vi "loadBoard.vi"(8 "error in (no error)":errorcluster, 10 "continuous":bool, 11 "SpinCore in":refnum<class "SpinCore.lvclass">) -> (0 "error out":errorcluster, 3 "SpinCore out":refnum<class "SpinCore.lvclass">)   [LabVIEW 2011, in "Hardware.lvlib" / "Channels.lvlib" / "SpinCore.lvclass"]
uses:
  SpinCore.lvclass
  SpinCore.lvclass/SpinCore.ctl
panel:
  out "Instructions":T1(array[cluster]) {"Op Code" items=["Continue", "Stop", "Loop", "End Loop", "JSR", "RTS", "Branch", "Long Delay", "Wait"]; "Amp Register2" items=["0", "1", "2", "3"]; "Phase Register2" items=["0", "1", "2", "3", "4", "5", "6", "7", "8", "9", "10", "11", "12", "13", "14", "15"]; "Freq Register2" items=["0", "1", "2", "3", "4", "5", "6", "7", "8", "9", "10", "11", "12", "13", "14", "15"]; "Amp Register1" items=["0", "1", "2", "3"]; "Phase Register1" items=["0", "1", "2", "3", "4", "5", "6", "7", "8", "9", "10", "11", "12", "13", "14", "15"]; "Freq Register1" items=["0", "1", "2", "3", "4", "5", "6", "7", "8", "9", "10", "11", "12", "13", "14", "15"]; "Length" format="%.6p"}
  out "dataChannel1":dbl[][](array[numeric])
  out "dataChannel0":dbl[][](array[numeric])
  # "0"
  # "1"
  # "2"
  # "3"
  # "4"
  # "5"
  # "6"
  # "7"
  # "8"
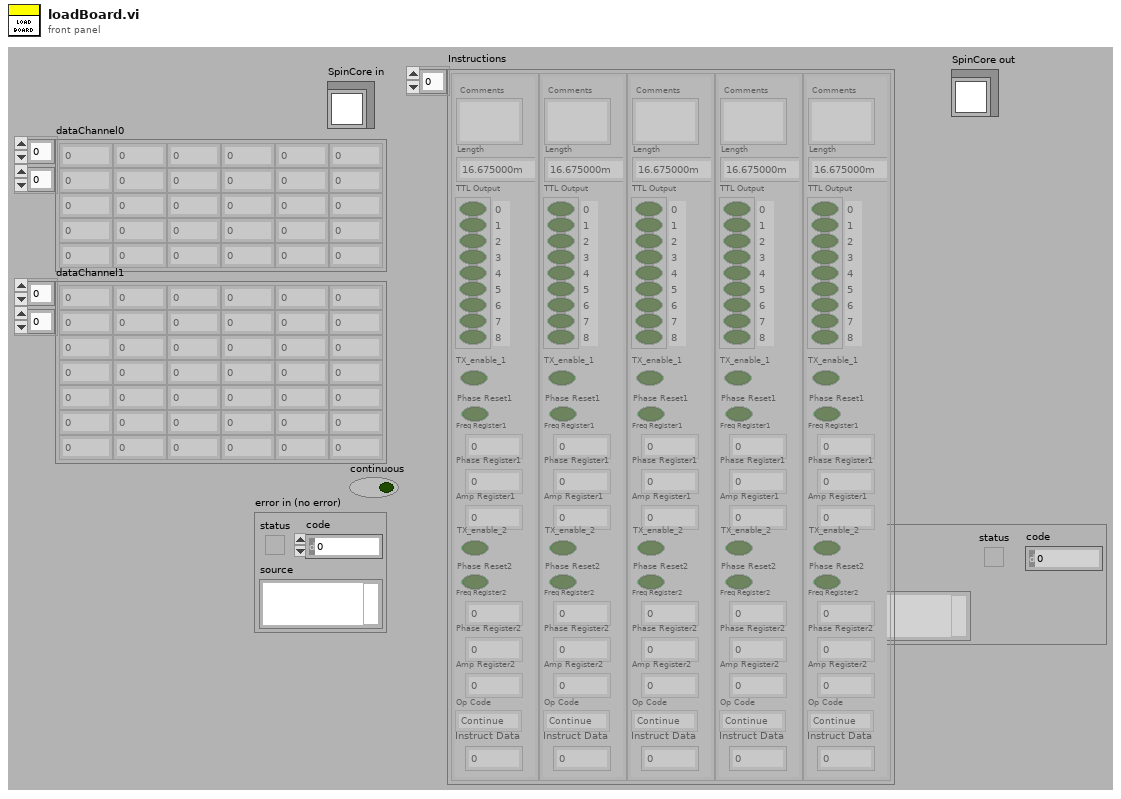
[diagram p1: front panel]
types:
  T1 = cluster{"Comments":string, "Length":dbl, "TTL Output":bool[], "TX_enable_1":bool, "Phase Reset1":bool, "Freq Register1":i32, "Phase Register1":i32, "Amp Register1":i32, "TX_enable_2":bool, "Phase Reset2":bool, "Freq Register2":i32, "Phase Register2":i32, "Amp Register2":i32, "Instruct Data":i32, "Op Code":i32}[]
  T2 = enum16{"Pulse Program", "Frequency Registers", "TX Phase Registers", "RX Phase Registers"}
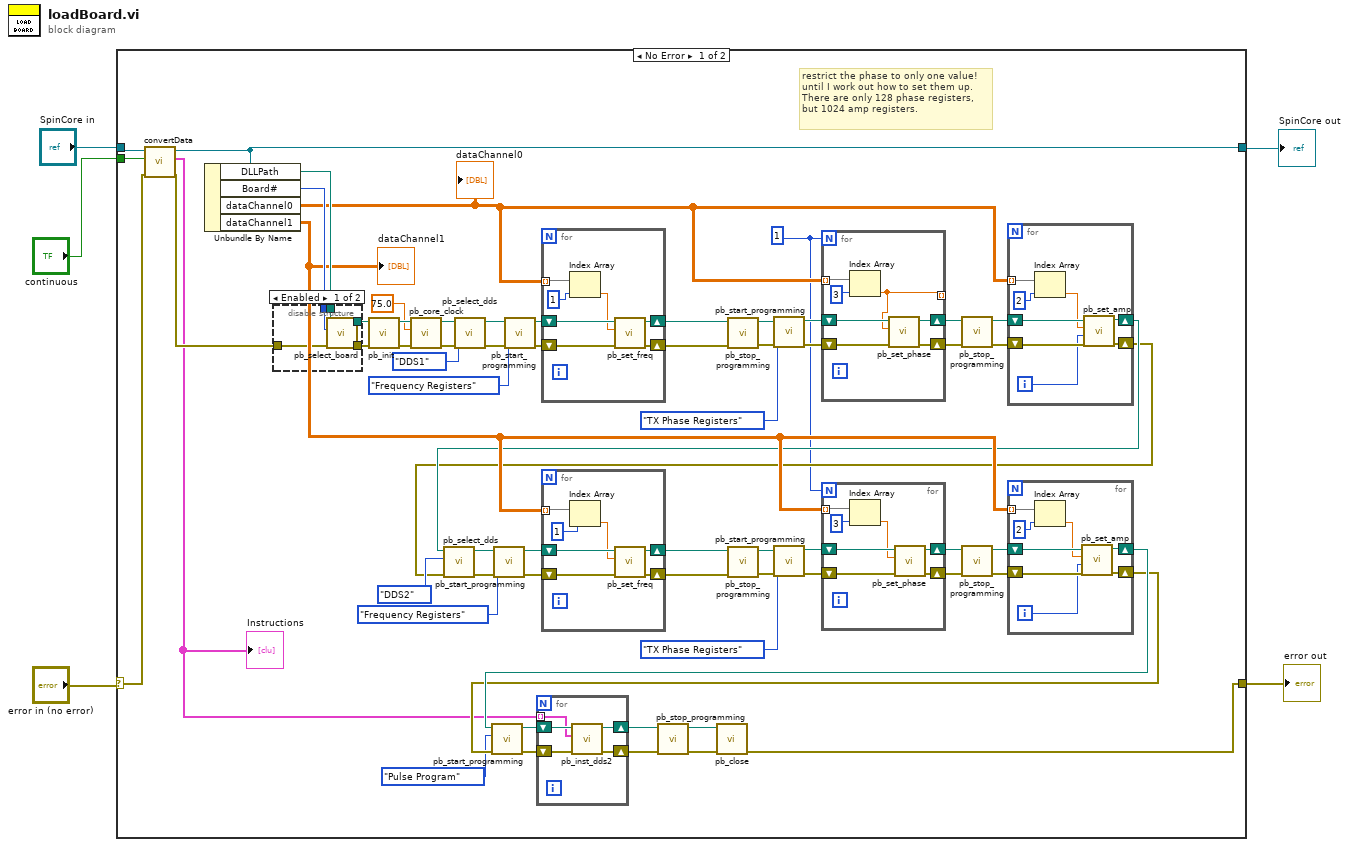
[diagram p0: block diagram]
diagram:
  n1 = case shown="No Error" "error in (no error)" {
    selector: "error in (no error)" -> [w16 w127]
    tunnel: [w19 w127] -> w4
    tunnel: [w17 w126] -> w2
    tunnel: "SpinCore in" -> [w18 w126]
    tunnel: "continuous" -> [w7 _]
    frame No Error {
      w6 = 1
      # "restrict the phase to only one value!\nuntil I work out how to set them up.\nThere are only 128 phase registers,\nbut 1024 amp registers."
      n2 = call "convertData.vi"("error in (no error)"=w16, "continuous"=w7, "SpinCore in"=w18) -> ("error out"=w15:errorcluster, "Instructions"=w14:T1, "SpinCore out"=w17:refnum<class "SpinCore.lvclass">)  [unwired: 6 in]
      "Instructions" <- w14
      n3 = Unbundle By Name(w17) -> ("DLLPath"=w50:path, "Board#"=w51:i32, "dataChannel0"=w33:dbl[][], "dataChannel1"=w32:dbl[][])
      "dataChannel0" <- w33
      "dataChannel1" <- w32
      n4 = disable-structure shown="Enabled" {
        disable-tunnel: [w74 w76] -> w69
        disable-tunnel: w51 -> [w73 _]
        disable-tunnel: w50 -> [w72 w76]
        disable-tunnel: w15 -> [w71 w75]
        disable-tunnel: [w70 w75] -> w8
        frame Enabled {
          n5 = call <userlib>:"pb_select_board.vi"("error in (no error)"=w71, "board_num"=w73, "path in"=w72) -> ("error out"=w70:errorcluster, "path out"=w74:path)  [unwired: 7 in]
        }
        frame Disabled {
        }
      }
      n6 = call <userlib>:"pb_init.vi"("error in (no error)"=w8, "path in"=w69) -> ("error out"=w11:errorcluster, "path out"=w12:path)  [unwired: 8 in]
      n7 = call <userlib>:"pb_core_clock.vi"("error in (no error)"=w11, "clock_freq (MHz)"=75.0, "path in"=w12) -> ("error out"=w10:errorcluster, "path out"=w13:path)  [unwired: 7 in]
      n8 = call <userlib>:"pb_select_dds.vi"("error in (no error)"=w10, "Device"=enum16{"DDS1", "DDS2"}."DDS1", "path in"=w13) -> ("error out"=w67:errorcluster, "path out"=w68:path)  [unwired: 7 in]
      n9 = call <userlib>:"pb_start_programming.vi"("error in (no error)"=w67, "Device"=T2."Frequency Registers", "path in"=w68) -> ("error out"=w63:errorcluster, "path out"=w64:path)  [unwired: 7 in]
      n10 = for {
        shift-right: [w124] -> w61
        shift-left: w64 -> [w125]
        shift-right: [w122] -> w62
        shift-left: w63 -> [w123]
        tunnel: w33 -> [w121] mode=indexing
        n11 = Index Array(array=w121, index=1) -> (element=w119:dbl)
        n12 = call <userlib>:"pb_set_freq.vi"("error in (no error)"=w123, "freq (MHz)"=w119, "path in"=w125) -> ("error out"=w122:errorcluster, "path out"=w124:path)  [unwired: 7 in]
      }
      n13 = call <userlib>:"pb_stop_programming.vi"("error in (no error)"=w62, "path in"=w61) -> ("error out"=w55:errorcluster, "path out"=w56:path)  [unwired: 8 in]
      n14 = call <userlib>:"pb_start_programming.vi"("error in (no error)"=w55, "Device"=T2."TX Phase Registers", "path in"=w56) -> ("error out"=w59:errorcluster, "path out"=w60:path)  [unwired: 7 in]
      n15 = for {
        N: w6 -> [_]
        shift-right: [w115] -> w57
        shift-left: w60 -> [w116]
        shift-right: [w114] -> w58
        shift-left: w59 -> [w113]
        tunnel: w33 -> [w118] mode=indexing
        tunnel: [w112] -> _ mode=indexing
        n16 = Index Array(array=w118, index=3) -> (element=w112:dbl)
        n17 = call <userlib>:"pb_set_phase.vi"("error in (no error)"=w113, "phase (deg)"=w112, "path in"=w116) -> ("error out"=w114:errorcluster, "path out"=w115:path)  [unwired: 7 in]
      }
      n18 = call <userlib>:"pb_stop_programming.vi"("error in (no error)"=w58, "path in"=w57) -> ("error out"=w53:errorcluster, "path out"=w52:path)  [unwired: 8 in]
      n19 = for {
        tunnel: w33 -> [w109] mode=indexing
        shift-right: [w105] -> w29
        shift-left: w53 -> [w111]
        shift-right: [w106] -> w30
        shift-left: w52 -> [w110]
        i -> [w107]
        n20 = Index Array(array=w109, index=2) -> (element=w104:dbl)
        n21 = call <userlib>:"pb_set_amp.vi"("error in (no error)"=w111, "register"=w107, "amplitude (0-1)"=w104, "path in"=w110) -> ("error out"=w105:errorcluster, "path out"=w106:path)  [unwired: 6 in]
      }
      n22 = call <userlib>:"pb_select_dds.vi"("error in (no error)"=w29, "Device"=enum16{"DDS1", "DDS2"}."DDS2", "path in"=w30) -> ("error out"=w48:errorcluster, "path out"=w49:path)  [unwired: 7 in]
      n23 = call <userlib>:"pb_start_programming.vi"("error in (no error)"=w48, "Device"=T2."Frequency Registers", "path in"=w49) -> ("error out"=w45:errorcluster, "path out"=w46:path)  [unwired: 7 in]
      n24 = for {
        shift-right: [w102] -> w43
        shift-left: w46 -> [w103]
        shift-right: [w100] -> w44
        shift-left: w45 -> [w101]
        tunnel: w32 -> [w98] mode=indexing
        n25 = Index Array(array=w98, index=1) -> (element=w99:dbl)
        n26 = call <userlib>:"pb_set_freq.vi"("error in (no error)"=w101, "freq (MHz)"=w99, "path in"=w103) -> ("error out"=w100:errorcluster, "path out"=w102:path)  [unwired: 7 in]
      }
      n27 = call <userlib>:"pb_stop_programming.vi"("error in (no error)"=w44, "path in"=w43) -> ("error out"=w37:errorcluster, "path out"=w38:path)  [unwired: 8 in]
      n28 = call <userlib>:"pb_start_programming.vi"("error in (no error)"=w37, "Device"=T2."TX Phase Registers", "path in"=w38) -> ("error out"=w41:errorcluster, "path out"=w42:path)  [unwired: 7 in]
      n29 = for {
        N: w6 -> [_]
        shift-right: [w95] -> w39
        shift-left: w42 -> [w96]
        shift-right: [w93] -> w40
        shift-left: w41 -> [w94]
        tunnel: w32 -> [w91] mode=indexing
        n30 = Index Array(array=w91, index=3) -> (element=w92:dbl)
        n31 = call <userlib>:"pb_set_phase.vi"("error in (no error)"=w94, "phase (deg)"=w92, "path in"=w96) -> ("error out"=w93:errorcluster, "path out"=w95:path)  [unwired: 7 in]
      }
      n32 = call <userlib>:"pb_stop_programming.vi"("error in (no error)"=w40, "path in"=w39) -> ("error out"=w35:errorcluster, "path out"=w34:path)  [unwired: 8 in]
      n33 = for {
        tunnel: w32 -> [w87] mode=indexing
        shift-right: [w82] -> w27
        shift-left: w35 -> [w89]
        shift-right: [w83] -> w28
        shift-left: w34 -> [w88]
        i -> [w84]
        n34 = Index Array(array=w87, index=2) -> (element=w85:dbl)
        n35 = call <userlib>:"pb_set_amp.vi"("error in (no error)"=w89, "register"=w84, "amplitude (0-1)"=w85, "path in"=w88) -> ("error out"=w82:errorcluster, "path out"=w83:path)  [unwired: 6 in]
      }
      n36 = call <userlib>:"pb_start_programming.vi"("error in (no error)"=w27, "Device"=T2."Pulse Program", "path in"=w28) -> ("error out"=w25:errorcluster, "path out"=w24:path)  [unwired: 7 in]
      n37 = for {
        shift-right: [w80] -> w23
        shift-left: w24 -> [w78]
        shift-right: [w79] -> w22
        shift-left: w25 -> [w81]
        tunnel: w14 -> [w77] mode=indexing
        n38 = call <userlib>:"pb_inst_dds2.vi"("error in (no error)"=w81, "DDS-II Instruction"=w77, "path in"=w78) -> ("error out"=w79:errorcluster, "path out"=w80:path)  [unwired: 7 in]
      }
      n39 = call <userlib>:"pb_stop_programming.vi"("error in (no error)"=w22, "path in"=w23) -> ("error out"=w21:errorcluster, "path out"=w20:path)  [unwired: 8 in]
      n40 = call <userlib>:"pb_close.vi"("error in (no error)"=w21, "path in"=w20) -> ("error out"=w19:errorcluster)  [unwired: 8 in, 1 out]
    }
    frame Error {
    }
  }
  "error out" <- w4
  "SpinCore out" <- w2
